vi "XNET.Settings.vi"(6 "Action":enum8{"Get", "Set"}(ring), 8 "error in (no error)":errorcluster, 10 "XNET Settings":T1={"Database"="", "Cluster"="", "Port"="", "Baud rate [Bd]"=500000, "Termination"=1, "CAN I/O Mode"=0, "FD Baud rate [Bd]"=500000, "Priority"=100, "Use Legacy"=FALSE, "FD ISO Mode"=0, "Default Max Counter Value"=0.0, "Default Protect Type"=enum."Arb ID + Bytes Checksum with Inversion"} {"FD ISO Mode" items=["ISO", "Non ISO", "ISO Legacy"]; "CAN I/O Mode" items=["CAN 2.0", "CAN FD", "CAN FD+BRS"]; "Termination" items=["Off", "On"]}, 11 "Parent Ref in":T3 format="%.0x") -> (0 "error out":errorcluster, 2 "XNET Settings":T1={"Database"="", "Cluster"="", "Port"="", "Baud rate [Bd]"=500000, "Termination"=1, "CAN I/O Mode"=0, "FD Baud rate [Bd]"=500000, "Priority"=100, "Use Legacy"=FALSE, "FD ISO Mode"=0, "Default Max Counter Value"=0.0, "Default Protect Type"=enum."Arb ID + Bytes Checksum with Inversion"} {"FD ISO Mode" items=["ISO", "Non ISO", "ISO Legacy"]; "CAN I/O Mode" items=["CAN 2.0", "CAN FD", "CAN FD+BRS"]; "Termination" items=["Off", "On"]}, 3 "Item Ref out":T3 format="%.0x")   [LabVIEW 2025, in "Protection and Counter Addon System Explorer.lvlib"]
uses:
  Protection and Counter Addon System Explorer.lvlib
  Addon Shared/Types/XNET Settings.ctl
  SubModules/Frame-Protection-Support/Source/Shared/Types/Protection Type.ctl
  <vilib>/NI VeriStand/Custom Device API/Custom Device Item Ref.ctl
  Addon Shared/SubVIs/GUID Lookup.vi
  <vilib>/NI/NI VeriStand Advanced SysDef API/_SubVIs/SysDef.Property.Set.String.vi
  <vilib>/NI/NI VeriStand Advanced SysDef API/_SubVIs/SysDef.Property.Set.U64.vi
  <vilib>/NI/NI VeriStand Advanced SysDef API/_SubVIs/SysDef.Property.Set.U32.vi
  <vilib>/NI/NI VeriStand Advanced SysDef API/_SubVIs/SysDef.Property.Set.Variant.vi
  <vilib>/NI/NI VeriStand Advanced SysDef API/_SubVIs/SysDef.Property.Set.I32.vi
  <vilib>/NI/NI VeriStand Advanced SysDef API/_SubVIs/SysDef.Property.Set.Boolean.vi
  <vilib>/NI/NI VeriStand Advanced SysDef API/_SubVIs/SysDef.Property.Set.DBL.vi
  <vilib>/NI VeriStand/Custom Device API/Get Item Property (String).vi
  <vilib>/NI VeriStand/Custom Device API/Get Item Property (U64).vi
  <vilib>/NI VeriStand/Custom Device API/Get Item Property (U32).vi
  <vilib>/NI VeriStand/Custom Device API/Get Item Property (Variant).vi
  <vilib>/NI VeriStand/Custom Device API/Get Item Property (I32).vi
  <vilib>/NI VeriStand/Custom Device API/Get Item Property (Boolean).vi
  <vilib>/NI VeriStand/Custom Device API/Get Item Property (Double).vi
  <vilib>/NI VeriStand/Custom Device API/Custom Device API.lvlib
  <vilib>/NI/NI VeriStand Advanced SysDef API/SysDef API/Advanced System Definition.lvlib
  Addon Shared/Protection and Counter Addon Shared.lvlib
  SubModules/Frame-Protection-Support/Source/Shared/Protection and Counter Support Shared.lvlib
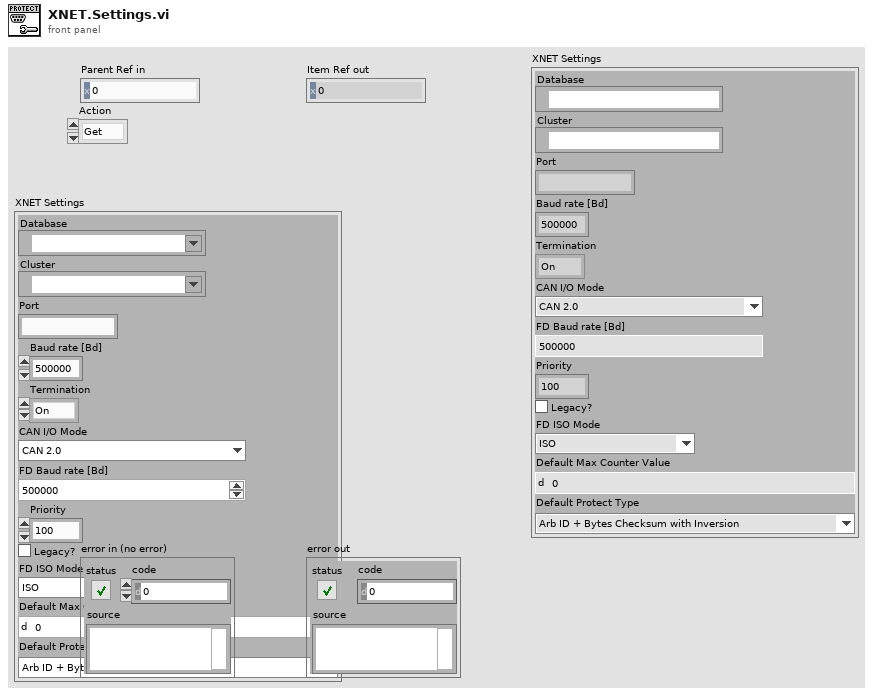
[diagram p1: front panel]
types:
  T1 = typedef "Protection and Counter Addon Shared.lvlib/XNET Settings.ctl" = cluster{"Database":refnum<k21>, "Cluster":refnum<k21>, "Port":string, "Baud rate [Bd]":u64, "Termination":u32, "CAN I/O Mode":u32, "FD Baud rate [Bd]":u64, "Priority":i32, "Use Legacy":bool, "FD ISO Mode":u32, "Default Max Counter Value":dbl, "Default Protect Type":T2}
  T2 = typedef "Protection and Counter Support Shared.lvlib/Protection Type.ctl" = enum16{"Arb ID + Bytes Checksum with Inversion", "Arb ID + Bytes CRC with Inversion", "Reversed Raw Signal Checksum with Inversion", "Concatenated Two's Compliment"}
  T3 = typedef "Custom Device API.lvlib/Custom Device Item Ref.ctl" = u64
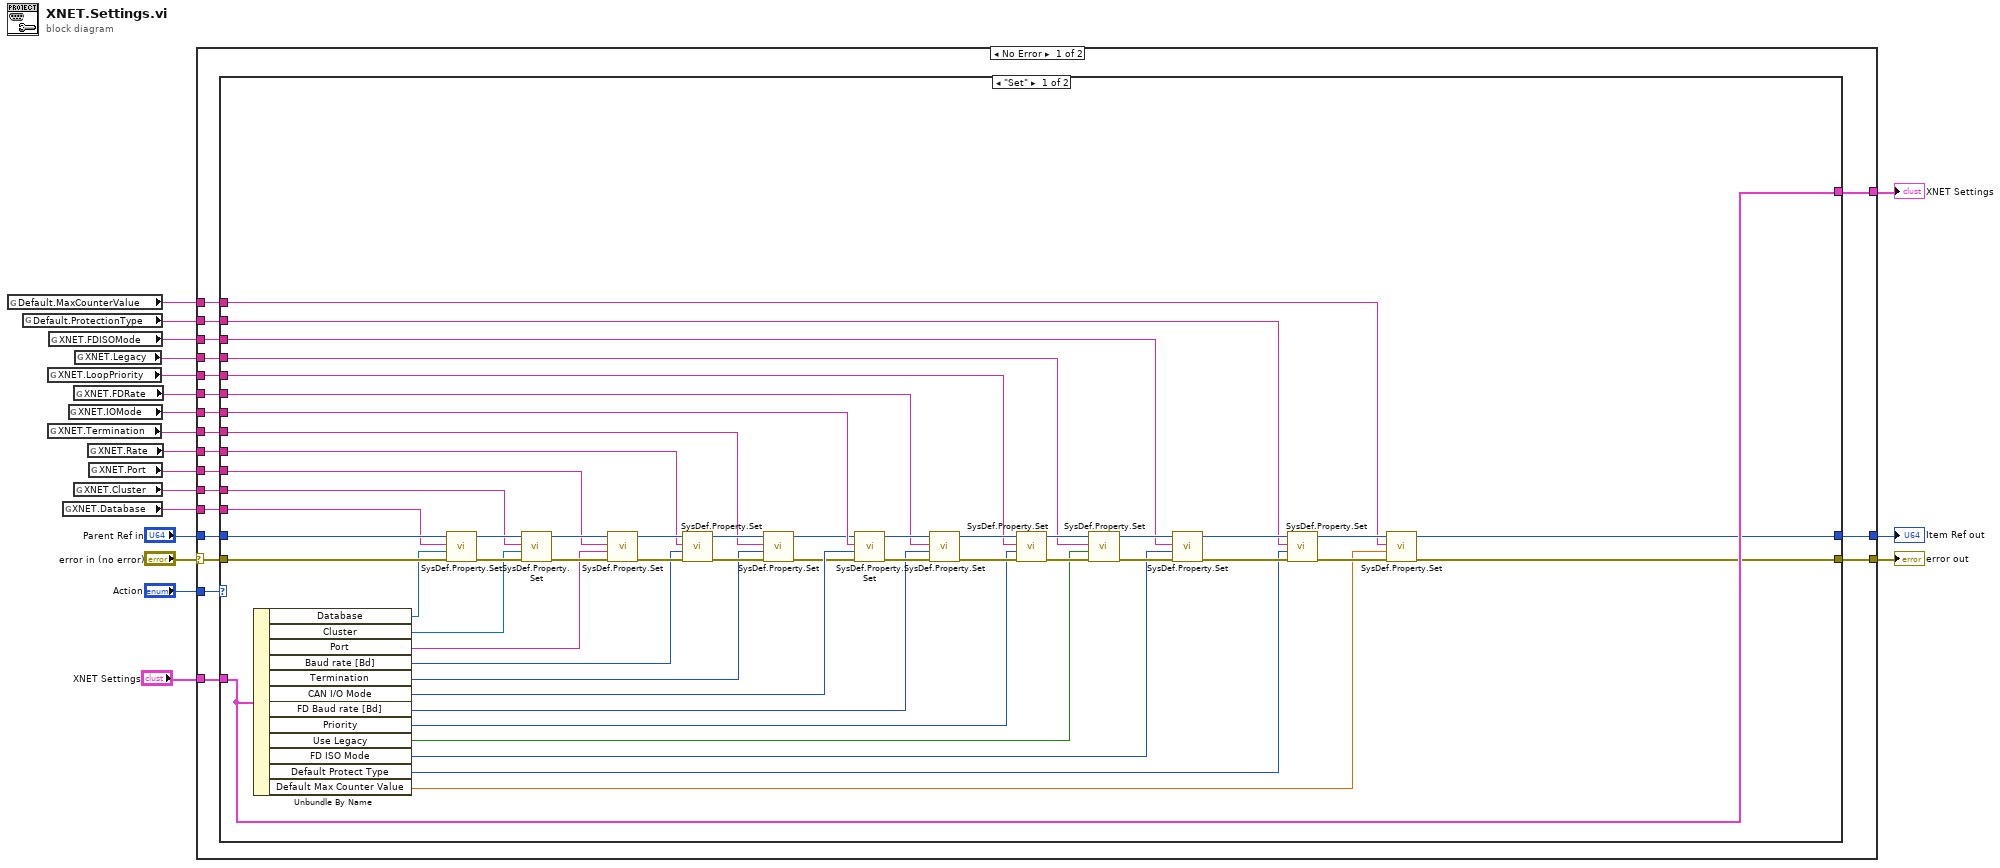
[diagram p0: block diagram]
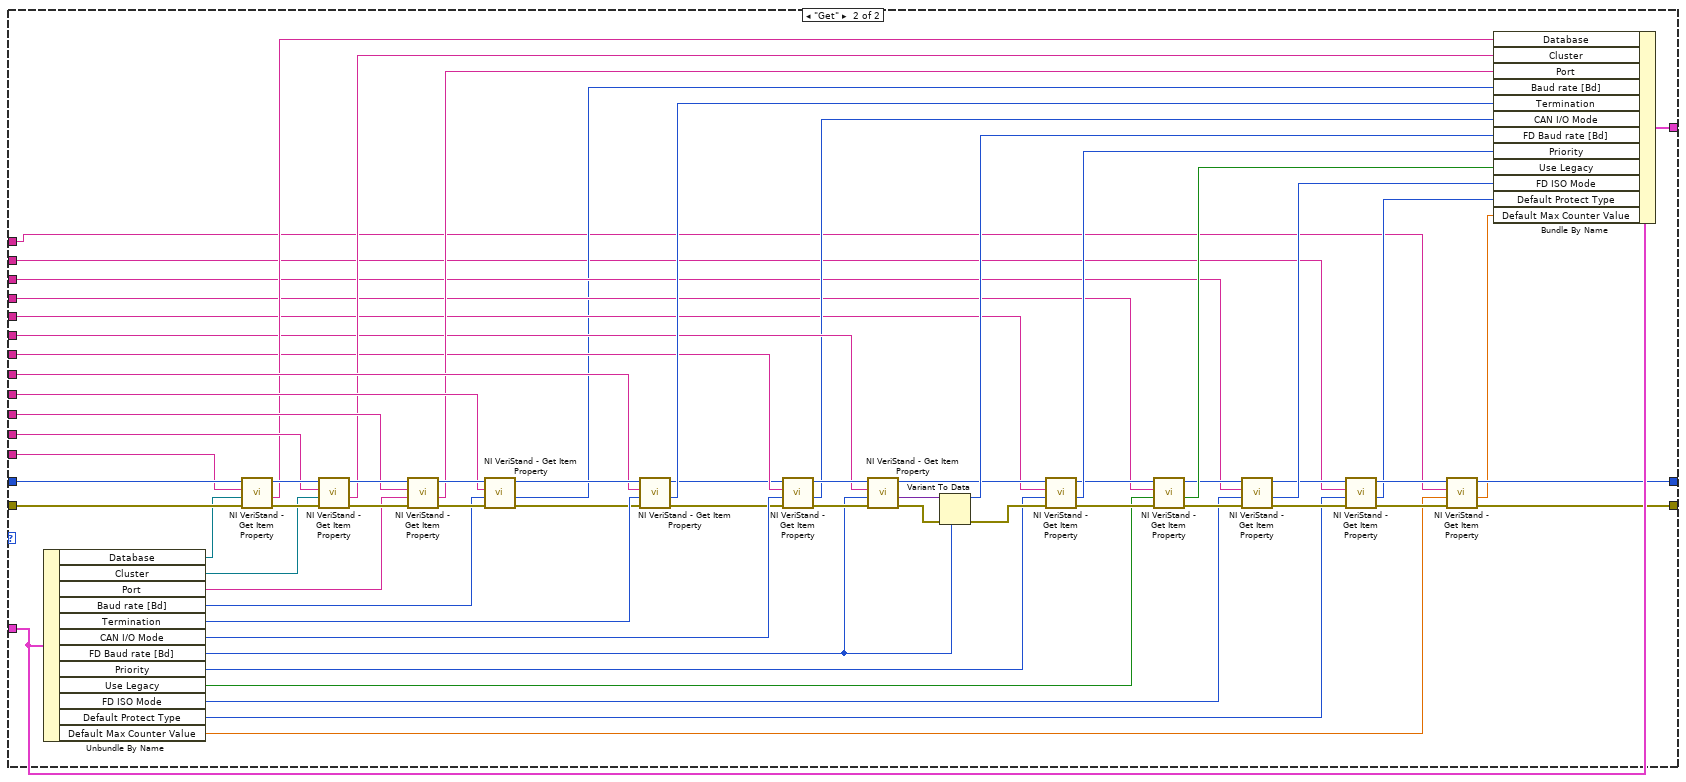
[diagram p2: hidden frame]
diagram:
  n1 = global read "GUID Lookup.vi" "Default.MaxCounterValue"() -> (w2:string)
  n2 = global read "GUID Lookup.vi" "Default.ProtectionType"() -> (w1:string)
  n3 = global read "GUID Lookup.vi" "XNET.LoopPriority"() -> (w5:string)
  n4 = global read "GUID Lookup.vi" "XNET.Termination"() -> (w8:string)
  n5 = global read "GUID Lookup.vi" "XNET.FDISOMode"() -> (w3:string)
  n6 = global read "GUID Lookup.vi" "XNET.Database"() -> (w12:string)
  n7 = global read "GUID Lookup.vi" "XNET.IOMode"() -> (w7:string)
  n8 = global read "GUID Lookup.vi" "XNET.FDRate"() -> (w6:string)
  n9 = global read "GUID Lookup.vi" "XNET.Cluster"() -> (w11:string)
  n10 = global read "GUID Lookup.vi" "XNET.Legacy"() -> (w4:string)
  n11 = global read "GUID Lookup.vi" "XNET.Rate"() -> (w9:string)
  n12 = global read "GUID Lookup.vi" "XNET.Port"() -> (w10:string)
  n13 = case shown="No Error" "error in (no error)" {
    selector: "error in (no error)" -> [w29 w158]
    tunnel: "Parent Ref in" -> [w38 w157]
    tunnel: w12 -> [w37 _]
    tunnel: "XNET Settings" -> [w36 w156]
    tunnel: [w35 w158] -> w17
    tunnel: [w34 w157] -> w16
    tunnel: w11 -> [w33 _]
    tunnel: w10 -> [w32 _]
    tunnel: w8 -> [w31 _]
    tunnel: w9 -> [w30 _]
    tunnel: "Action" -> [w28 _]
    tunnel: [w27 w156] -> w13
    tunnel: w7 -> [w26 _]
    tunnel: w6 -> [w25 _]
    tunnel: w5 -> [w24 _]
    tunnel: w4 -> [w23 _]
    tunnel: w3 -> [w22 _]
    tunnel: w2 -> [w21 _]
    tunnel: w1 -> [w20 _]
    frame No Error {
      n14 = case shown="\"Set\"" w28 {
        tunnel: w38 -> [w89 w155]
        tunnel: w37 -> [w88 w154]
        tunnel: w36 -> [w70 w137]
        tunnel: [w45 w96] -> w35
        tunnel: [w44 w97] -> w34
        tunnel: w33 -> [w75 w146]
        tunnel: w32 -> [w74 w145]
        tunnel: w31 -> [w73 w144]
        tunnel: w30 -> [w72 w143]
        tunnel: w29 -> [w71 w142]
        tunnel: [w70 w132] -> w27
        tunnel: w26 -> [w66 w128]
        tunnel: w25 -> [w65 w127]
        tunnel: w24 -> [w57 w116]
        tunnel: w23 -> [w54 w110]
        tunnel: w22 -> [w50 w106]
        tunnel: w21 -> [w40 w93]
        tunnel: w20 -> [w39 w92]
        frame "Set" {
          n15 = Unbundle By Name(w70) -> ("Database"=w69:refnum<k21>, "Cluster"=w79:refnum<k21>, "Port"=w78:string, "Baud rate [Bd]"=w77:u64, "Termination"=w76:u32, "CAN I/O Mode"=w64:u32, "FD Baud rate [Bd]"=w63:u64, "Priority"=w58:i32, "Use Legacy"=w53:bool, "FD ISO Mode"=w49:u32, "Default Protect Type"=w42:T2, "Default Max Counter Value"=w41:dbl)
          n16 = call-poly <vilib>:"SysDef.Property.Set.vi"("error in (no error)"=w71, "Value"=w69, "Property Name"=w88, "nodeID"=w89) -> ("error out"=w85:errorcluster, "nodeID out"=w84:u64)  [unwired: 6 in]
          n17 = call-poly <vilib>:"SysDef.Property.Set.vi"("error in (no error)"=w85, "Value"=w79, "Property Name"=w75, "nodeID"=w84) -> ("error out"=w86:errorcluster, "nodeID out"=w87:u64)  [unwired: 6 in]
          n18 = call-poly <vilib>:"SysDef.Property.Set.vi"("error in (no error)"=w86, "Value"=w78, "Property Name"=w74, "nodeID"=w87) -> ("error out"=w81:errorcluster, "nodeID out"=w80:u64)  [unwired: 6 in]
          n19 = call-poly <vilib>:"SysDef.Property.Set.vi"("error in (no error)"=w81, "Value"=w77, "Property Name"=w72, "nodeID"=w80) -> ("error out"=w82:errorcluster, "nodeID out"=w83:u64)  [unwired: 6 in]
          n20 = call-poly <vilib>:"SysDef.Property.Set.vi"("error in (no error)"=w82, "Value"=w76, "Property Name"=w73, "nodeID"=w83) -> ("error out"=w62:errorcluster, "nodeID out"=w61:u64)  [unwired: 6 in]
          n21 = call-poly <vilib>:"SysDef.Property.Set.vi"("error in (no error)"=w62, "Value"=w64, "Property Name"=w66, "nodeID"=w61) -> ("error out"=w68:errorcluster, "nodeID out"=w67:u64)  [unwired: 6 in]
          n22 = call-poly <vilib>:"SysDef.Property.Set.vi"("error in (no error)"=w68, "Value"=w63, "Property Name"=w65, "nodeID"=w67) -> ("error out"=w60:errorcluster, "nodeID out"=w59:u64)  [unwired: 6 in]
          n23 = call-poly <vilib>:"SysDef.Property.Set.vi"("error in (no error)"=w60, "Value"=w58, "Property Name"=w57, "nodeID"=w59) -> ("error out"=w56:errorcluster, "nodeID out"=w55:u64)  [unwired: 6 in]
          n24 = call-poly <vilib>:"SysDef.Property.Set.vi"("error in (no error)"=w56, "Value"=w53, "Property Name"=w54, "nodeID"=w55) -> ("error out"=w52:errorcluster, "nodeID out"=w51:u64)  [unwired: 6 in]
          n25 = call-poly <vilib>:"SysDef.Property.Set.vi"("error in (no error)"=w52, "Value"=w49, "Property Name"=w50, "nodeID"=w51) -> ("error out"=w48:errorcluster, "nodeID out"=w47:u64)  [unwired: 6 in]
          n26 = call-poly <vilib>:"SysDef.Property.Set.vi"("error in (no error)"=w48, "Value"=w42, "Property Name"=w39, "nodeID"=w47) -> ("error out"=w46:errorcluster, "nodeID out"=w43:u64)  [unwired: 6 in]
          n27 = call-poly <vilib>:"SysDef.Property.Set.vi"("error in (no error)"=w46, "Value"=w41, "Property Name"=w40, "nodeID"=w43) -> ("error out"=w45:errorcluster, "nodeID out"=w44:u64)  [unwired: 6 in]
        }
        frame "Get" {
          n28 = Unbundle By Name(w137) -> ("Database"=w141:refnum<k21>, "Cluster"=w140:refnum<k21>, "Port"=w139:string, "Baud rate [Bd]"=w119:u64, "Termination"=w138:u32, "CAN I/O Mode"=w129:u32, "FD Baud rate [Bd]"=w124:u64, "Priority"=w115:i32, "Use Legacy"=w109:bool, "FD ISO Mode"=w105:u32, "Default Protect Type"=w90:T2, "Default Max Counter Value"=w91:dbl)
          n29 = call-poly <vilib>:"NI VeriStand - Get Item Property.vi"("error in (no error)"=w142, "Default Value"=w141, "Property Name"=w154, "Item Ref in"=w155) -> ("error out"=w151:errorcluster, "Value"=w136:string, "Item Ref out"=w150:T3)  [unwired: 4 in, 1 out]
          n30 = call-poly <vilib>:"NI VeriStand - Get Item Property.vi"("error in (no error)"=w151, "Default Value"=w140, "Property Name"=w146, "Item Ref in"=w150) -> ("error out"=w152:errorcluster, "Value"=w135:string, "Item Ref out"=w153:T3)  [unwired: 4 in, 1 out]
          n31 = call-poly <vilib>:"NI VeriStand - Get Item Property.vi"("error in (no error)"=w152, "Default Value"=w139, "Property Name"=w145, "Item Ref in"=w153) -> ("error out"=w148:errorcluster, "Value"=w134:string, "Item Ref out"=w147:T3)  [unwired: 4 in, 1 out]
          n32 = call-poly <vilib>:"NI VeriStand - Get Item Property.vi"("error in (no error)"=w148, "Default Value"=w119, "Property Name"=w143, "Item Ref in"=w147) -> ("error out"=w103:errorcluster, "Value"=w102:u64, "Item Ref out"=w149:T3)  [unwired: 4 in, 1 out]
          n33 = call-poly <vilib>:"NI VeriStand - Get Item Property.vi"("error in (no error)"=w103, "Default Value"=w138, "Property Name"=w144, "Item Ref in"=w149) -> ("error out"=w120:errorcluster, "Value"=w133:u32, "Item Ref out"=w121:T3)  [unwired: 4 in, 1 out]
          n34 = call-poly <vilib>:"NI VeriStand - Get Item Property.vi"("error in (no error)"=w120, "Default Value"=w129, "Property Name"=w128, "Item Ref in"=w121) -> ("error out"=w131:errorcluster, "Value"=w126:u32, "Item Ref out"=w130:T3)  [unwired: 4 in, 1 out]
          n35 = call-poly <vilib>:"NI VeriStand - Get Item Property.vi"("error in (no error)"=w131, "Default Value"=w124, "Property Name"=w127, "Item Ref in"=w130) -> ("error out"=w123:errorcluster, "Value"=w125:variant, "Item Ref out"=w117:T3)  [unwired: 4 in, 1 out]
          n36 = Variant To Data(error in=w123, type=w124, Variant=w125) -> (data=w122:u64, error out=w118:errorcluster)
          n37 = call-poly <vilib>:"NI VeriStand - Get Item Property.vi"("error in (no error)"=w118, "Default Value"=w115, "Property Name"=w116, "Item Ref in"=w117) -> ("error out"=w113:errorcluster, "Value"=w114:i32, "Item Ref out"=w112:T3)  [unwired: 4 in, 1 out]
          n38 = call-poly <vilib>:"NI VeriStand - Get Item Property.vi"("error in (no error)"=w113, "Default Value"=w109, "Property Name"=w110, "Item Ref in"=w112) -> ("error out"=w108:errorcluster, "Value"=w111:bool, "Item Ref out"=w107:T3)  [unwired: 4 in, 1 out]
          n39 = call-poly <vilib>:"NI VeriStand - Get Item Property.vi"("error in (no error)"=w108, "Default Value"=w105, "Property Name"=w106, "Item Ref in"=w107) -> ("error out"=w100:errorcluster, "Value"=w104:u32, "Item Ref out"=w101:T3)  [unwired: 4 in, 1 out]
          n40 = call-poly <vilib>:"NI VeriStand - Get Item Property.vi"("error in (no error)"=w100, "Default Value"=w90, "Property Name"=w92, "Item Ref in"=w101) -> ("error out"=w99:errorcluster, "Value"=w94:u32, "Item Ref out"=w98:T3)  [unwired: 4 in, 1 out]
          n41 = call-poly <vilib>:"NI VeriStand - Get Item Property.vi"("error in (no error)"=w99, "Default Value"=w91, "Property Name"=w93, "Item Ref in"=w98) -> ("error out"=w96:errorcluster, "Value"=w95:dbl, "Item Ref out"=w97:T3)  [unwired: 4 in, 1 out]
          n42 = Bundle By Name(cluster=w137, "Database"=w136, "Cluster"=w135, "Port"=w134, "Baud rate [Bd]"=w102, "Termination"=w133, "CAN I/O Mode"=w126, "FD Baud rate [Bd]"=w122, "Priority"=w114, "Use Legacy"=w111, "FD ISO Mode"=w104, "Default Protect Type"=w94, "Default Max Counter Value"=w95) -> (w132:T1)
        }
      }
    }
    frame Error {
    }
  }
  "Item Ref out" <- w16
  "error out" <- w17
  "XNET Settings" <- w13
